vi "Start Polling Core.vi"(8 "Error In":errorcluster, 11 "CS++BaseActor in":refnum<class "CS++BaseActor.lvclass">) -> (0 "Error Out":errorcluster, 3 "CS++BaseActor out":refnum<class "CS++BaseActor.lvclass">)   [LabVIEW 2015, in "CS++BaseActor.lvlib" / "CS++BaseActor.lvclass"]
doc: "Start polling if polling intervall is less equal 0s."
uses:
  CS++BaseActor.lvclass
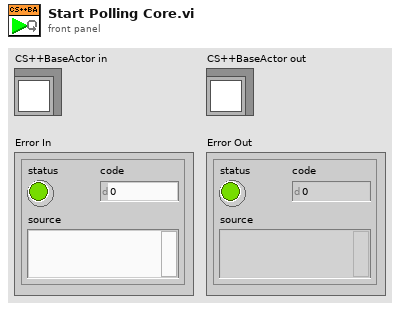
[diagram p1: front panel]
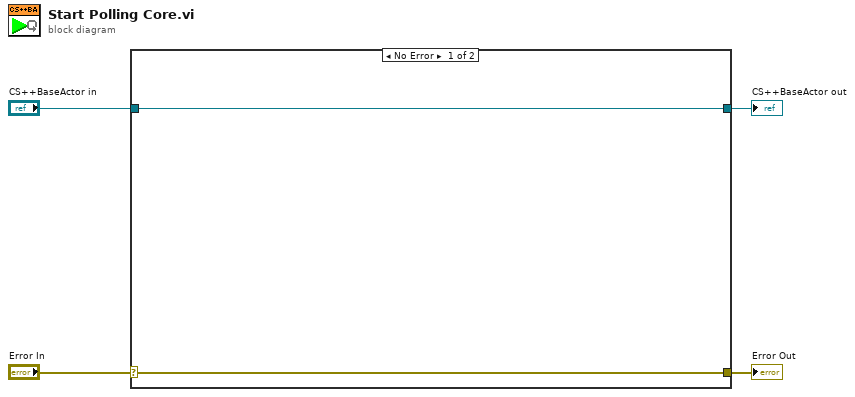
[diagram p0: block diagram]
diagram:
  n1 = case shown="No Error" "Error In" {
    selector: "Error In" -> [w6 w8]
    tunnel: [w6 w8] -> w3
    tunnel: [w5 w7] -> w1
    tunnel: "CS++BaseActor in" -> [w5 w7]
    frame No Error {
    }
    frame Error {
    }
  }
  "Error Out" <- w3
  "CS++BaseActor out" <- w1
